vi "GetTandH.vi"(8 "error in (no error)":errorcluster, 11 "Temperhum.PCSensor in":refnum<class "Temperhum.PCSensor.lvclass">) -> (0 "error out":errorcluster, 1 "Humidity (%RH)":dbl, 2 "Temperature (K)":dbl, 3 "Temperhum.PCSensor out":refnum<class "Temperhum.PCSensor.lvclass">)   [LabVIEW 2019, in "Temperhum.PCSensor.lvclass"]
uses:
  Temperhum.PCSensor.lvclass
  Temperhum.PCSensor.lvclass/Temperhum.PCSensor.ctl
  drivers/TEMPerHUM/TEMPerHUM.lvlib
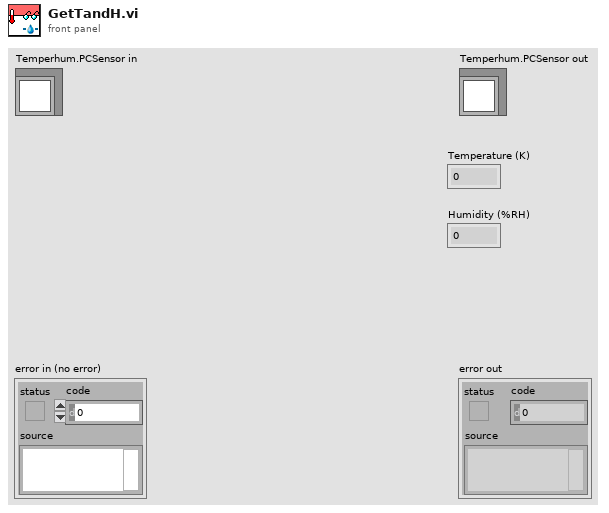
[diagram p1: front panel]
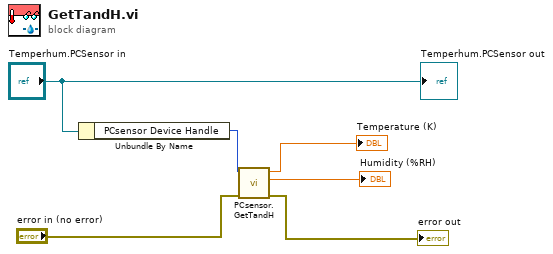
[diagram p0: block diagram]
diagram:
  n1 = Unbundle By Name("Temperhum.PCSensor in") -> ("PCsensor Device Handle"=w2:i64)
  n2 = call "PCsensor.GetTandH.vi"("error in (no error)"="error in (no error)", "PCsensor Device Handle"=w2) -> ("error out"=→"error out":errorcluster, "Humidity"=→"Humidity (%RH)":dbl, "Temperature"=→"Temperature (K)":dbl)  [unwired: 7 in]
  "Temperhum.PCSensor out" <- "Temperhum.PCSensor in"
